vi "isDST.vi"(2 "timestamp (now)":timestamp) -> (7 "is DST?":bool)   [LabVIEW 2013]
doc: "Timestamp is not converted to UTC time, so the year being evaluated is the year of the timestamp, not the current year at GMT."
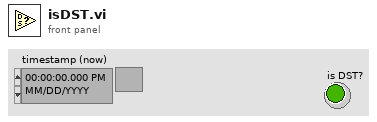
[diagram p1: front panel]
types:
  T1 = typedef "LVDateTimeRec.ctl" = cluster{"fractional second":dbl, "second":i32, "minute":i32, "hour":i32, "day of month":i32, "month":i32, "year":i32, "day of week":i32, "day of year":i32, "DST":i32}
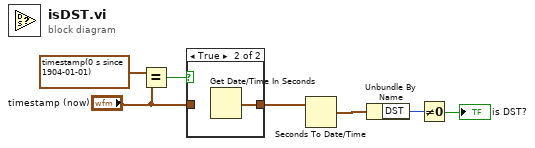
[diagram p0: block diagram]
diagram:
  n1 = Equal?(x=timestamp(0 s since 1904-01-01), y="timestamp (now)") -> (x = y?=w5:bool)
  n2 = case shown="True" w5 {
    tunnel: [w8 w9] -> w4
    tunnel: "timestamp (now)" -> [w8 _]
    frame False {
    }
    frame True {
      n3 = Get Date/Time In Seconds() -> (seconds since 1Jan1904=w9:timestamp)
    }
  }
  n4 = Seconds To Date/Time(time stamp (now)=w4) -> (date time rec=w7:T1)  [unwired: 1 in]
  n5 = Unbundle By Name(w7) -> ("DST"=w1:i32)
  n6 = Not Equal To 0?(x=w1) -> (x != 0?=→"is DST?":bool)
